vi "Measurement Logic.vi"() -> ()   [LabVIEW 2021, in "Line Transient Response with Pin Map.lvlib"]
uses:
  Line Transient Response with Pin Map.lvlib
  <vilib>/Plug-In SDKs/Measurements/Measure Call Context/Measure Call Context.lvclass
  Measurement Results.ctl
  Measurement Configuration.ctl
  <instrlib>/niScope/Controls/niScope vertical coupling.ctl
  subVIs/Reference values.ctl
  <vilib>/Plug-In SDKs/Clients/Session Management V1/Session Reservation/Session Reservation.lvclass
  common/builds/PMIC Common.lvlibp/Instrument Control/Scope/TClk/Instrument Info.ctl
  common/builds/PMIC Common.lvlibp/Instrument Control/Scope Parameters.ctl
  common/builds/PMIC Common.lvlibp/1abvi3w/instr.lib/niScope/Controls/niScope vertical coupling.ctl
  <instrlib>/niDCPower/nidcpower.llb/niDCPower Sense.ctl
  <instrlib>/niDCPower/nidcpower.llb/niDCPower Source Mode.ctl
  <instrlib>/niDCPower/nidcpower.llb/niDCPower Wait For Event - Event.ctl
  <instrlib>/niDCPower/nidcpower.llb/niDCPower Output Function.ctl
  <instrlib>/niDCPower/nidcpower.llb/niDCPower Aperture Time Units.ctl
  <vilib>/Plug-In SDKs/Measurements/Measure Call Context/Reserve Sessions - NPin.vi
  <vilib>/Plug-In SDKs/Sessions/niDCPower/Initialize Sessions - NSess.vi
  <vilib>/Plug-In SDKs/Sessions/niDCPower/Get Connections - 1Pin 1Conn.vi
  <instrlib>/niDCPower/nidcpower.llb/niDCPower Configure Digital Edge Measure Trigger With Channels.vi
  <instrlib>/niDCPower/nidcpower.llb/niDCPower Configure Digital Edge Source Trigger With Channels.vi
  <vilib>/Plug-In SDKs/Sessions/niScope/Initialize Sessions - NSess.vi
  <vilib>/Plug-In SDKs/Sessions/niScope/Get Connections - NPin MConn.vi
  <instrlib>/niScope/Configure/Trigger/niScope Configure Trigger Digital.vi
  <vilib>/Plug-In SDKs/Sessions/niDCPower/NI Session Management niDCPower.lvlib
  common/builds/PMIC Common.lvlibp
  <vilib>/Plug-In SDKs/Sessions/niScope/NI Session Management niScope.lvlib
panel:
  in  "measurement configuration":T1={"DUT setup time"=1.0, "Nominal output voltage"=3.3, "Source pin name"="", "Source current limit"=0.25, "Source maximum power"=300.0, "Source sample rate"=1800000.0, "Source voltage set point 1"=7.0, "Source voltage set point 2"=20.0, "Source voltatge pulse duration"=0.005, "Source voltage delay t1"=0.005, "Source voltage delay t2"=0.005, "Source voltage falling slew rate"=0.0055, "Source voltage rising slew rate"=24.0, "Source transient response"=1042, "Source voltage gain bandwidth"=2000.0, "Source voltage compensation frequency"=3530.0, "Source voltage pole-zero ratio"=2.0, "Load pin name"="", "Load voltage limit range"=4.0, "Load current level range"=4.0, "Load current level"=0.03, "Load transient response"=1042, "Load current gain bandwidth"=14000.0, "Load current compensation frequency"=180000.0, "Load current pole-zero ratio"=0.3, "Pin Names for Scope"=[], "vertical range"=[], "vertical offset"=[], "probe attenuation"=[], "vertical coupling"=[], "channel enabled"=[], "input impedance"=[], "max input frequency"=[], "min sample rate"=[], "reference position"=[], "min record length"=[], "enforce realtime"=[]} {"input impedance" items=["1 mega ohm"=0, "50 ohms"=2]; "vertical coupling" items=["AC", "DC", "Ground"]; "Source voltatge pulse duration" format="%#_6p"; "Source voltage rising slew rate" format="%#_6p"; "Load current pole-zero ratio" format="%#.2p"; "Load current compensation frequency" step=1000000.0 format="%#.2p"; "Load transient response" items=["Slow"=1041, "Normal"=1038, "Fast"=1039, "Custom"=1042]; "Source transient response" items=["Slow"=1041, "Normal"=1038, "Fast"=1039, "Custom"=1042]}
  out "measurement results":T3
  out "measure call context out":refnum<class "Measure Call Context.lvclass">
  in  "measure call context in":refnum<class "Measure Call Context.lvclass">
  out "error out":errorcluster
  in  "error in":errorcluster
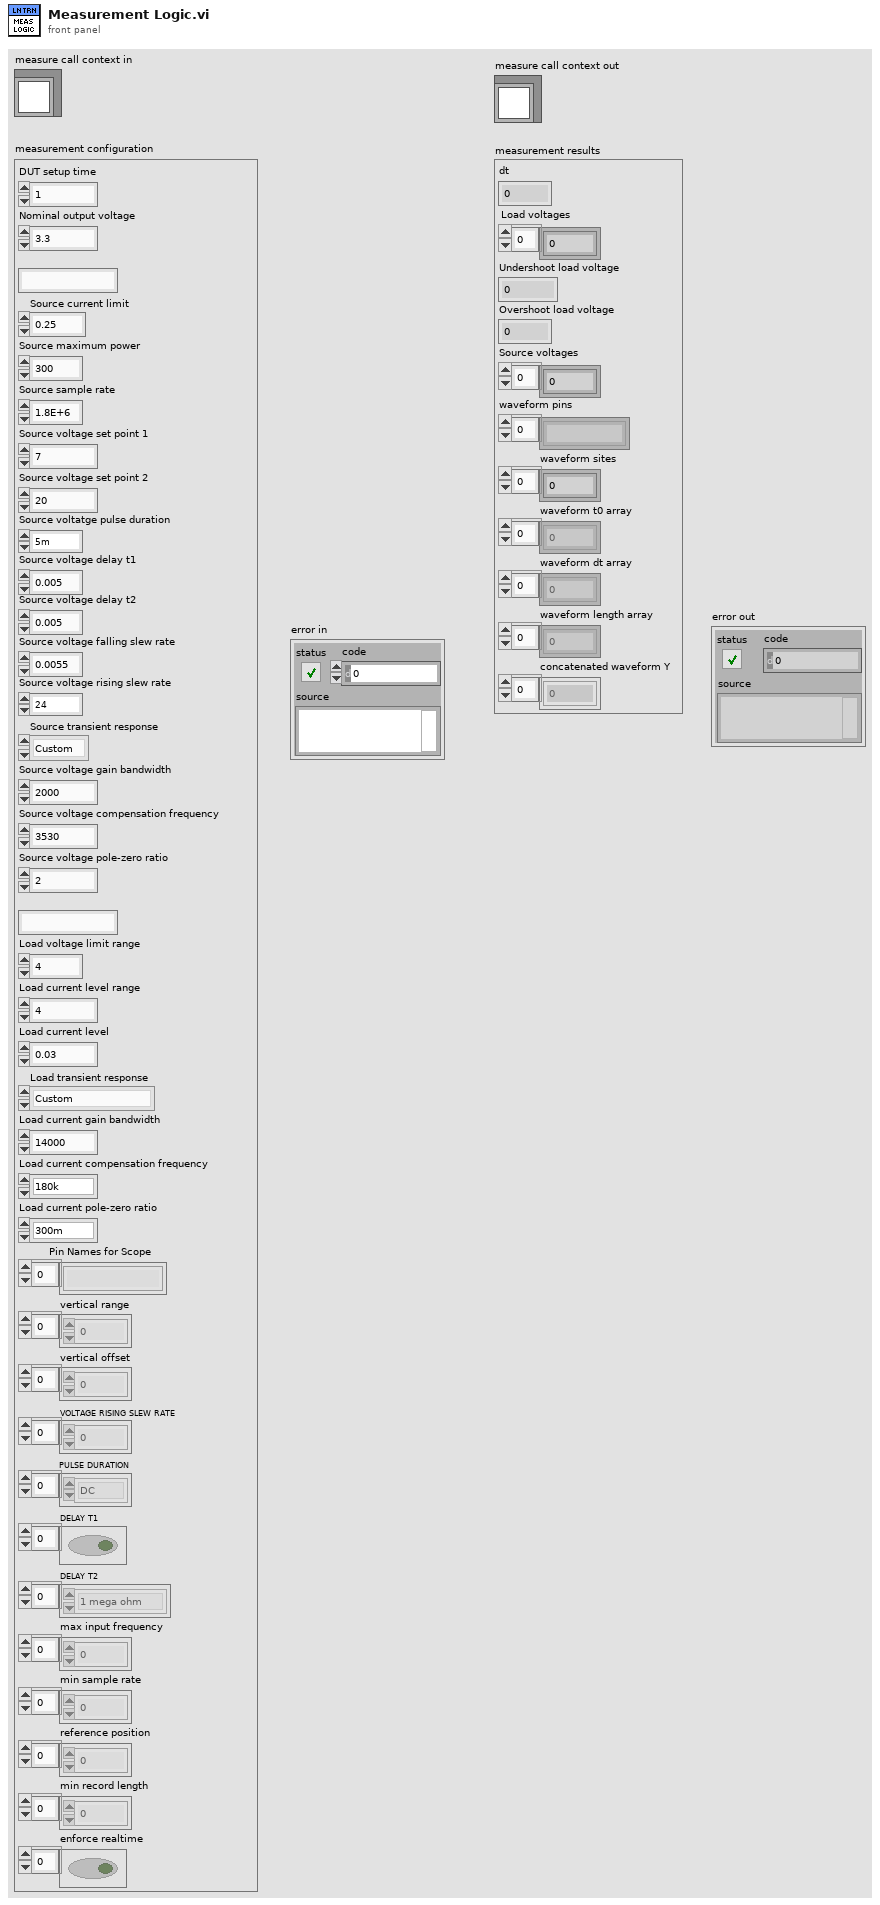
[diagram p1: front panel]
types:
  T1 = typedef "Line Transient Response with Pin Map.lvlib/Measurement Configuration.ctl" = cluster{"DUT setup time":dbl, "Nominal output voltage":dbl, "Source pin name":string, "Source current limit":dbl, "Source maximum power":dbl, "Source sample rate":dbl, "Source voltage set point 1":dbl, "Source voltage set point 2":dbl, "Source voltatge pulse duration":dbl, "Source voltage delay t1":dbl, "Source voltage delay t2":dbl, "Source voltage falling slew rate":dbl, "Source voltage rising slew rate":dbl, "Source transient response":i32, "Source voltage gain bandwidth":dbl, "Source voltage compensation frequency":dbl, "Source voltage pole-zero ratio":dbl, "Load pin name":string, "Load voltage limit range":dbl, "Load current level range":dbl, "Load current level":dbl, "Load transient response":i32, "Load current gain bandwidth":dbl, "Load current compensation frequency":dbl, "Load current pole-zero ratio":dbl, "Pin Names for Scope":string[], "vertical range":dbl[], "vertical offset":dbl[], "probe attenuation":dbl[], "vertical coupling":T2[], "channel enabled":bool[], "input impedance":u32[], "max input frequency":dbl[], "min sample rate":dbl[], "reference position":dbl[], "min record length":i32[], "enforce realtime":bool[]}
  T2 = typedef "niScope vertical coupling.ctl" = i32
  T3 = typedef "Line Transient Response with Pin Map.lvlib/Measurement Results.ctl" = cluster{"dt":dbl, "Load voltages":dbl[], "Undershoot load voltage":dbl, "Overshoot load voltage":dbl, "Source voltages":dbl[], "waveform pins":string[], "waveform sites":i32[], "waveform t0 array":dbl[], "waveform dt array":dbl[], "waveform length array":i32[], "concatenated waveform Y":dbl[]}
  T4 = typedef "Line Transient Response with Pin Map.lvlib/Reference values.ctl" = cluster{"dcpower session reservation":refnum<class "Session Reservation.lvclass">, "Source out":refnum<k15>, "Source channel name":string, "Load out":refnum<k15>, "Load channel name":string, "Scope out":refnum<k15>, "Scope channel name":string, "Source sequence name":string, "Source terminal name":string, "Start source terminal name":string, "Measure load terminal name":string, "Scope ref trigger source":string, "Measure record length smu":i32, "Aperture time":dbl, "Measure record length scope":i32, "scope session reservation":refnum<class "Session Reservation.lvclass">, "Scope handles":refnum<k15>[][], "connection map":map{string, T5[]}, "instrument info map array":map{string, cluster{"channel":string, "siteNumber":i32, "pin":string, "Scope Parameters":T6}[]}[], "Enable TClk":bool, "Number of records":i32, "measurement results":T3}
  T5 = typedef "PMIC Common.lvlibp/Instrument Info.ctl" = cluster{"instrument":string, "channel":string, "siteNumber":i32}
  T6 = typedef "PMIC Common.lvlibp/Scope Parameters.ctl" = cluster{"vertical range":dbl, "vertical offset":dbl, "probe attenuation":dbl, "vertical coupling":T7, "channel enabled":bool, "input impedance":u32, "maximum input frequency":dbl, "min sample rate":dbl, "reference position":dbl, "min record length":i32, "number of records":i32, "enforce realtime":bool}
  T7 = typedef "PMIC Common.lvlibp/niScope vertical coupling.ctl" = i32
  T8 = typedef "niDCPower Wait For Event - Event.ctl" = i32
  T9 = typedef "niDCPower Source Mode.ctl" = i32
  T10 = typedef "niDCPower Sense.ctl" = i32
  T11 = typedef "NI Session Management niDCPower.lvlib/Connection with Session.ctl" = cluster{"connection":T12, "session":refnum<k15>}
  T12 = typedef "NI Session Management V1 Client.lvlib/Session Reservation.lvclass/Connection.ctl" = cluster{"pin or relay name":string, "site":i32, "instrument type id":string, "channel":string}
  T13 = typedef "niDCPower Aperture Time Units.ctl" = i32
  T14 = typedef "niDCPower Output Function.ctl" = i32
  T15 = cluster{"Numeric":dbl, "Numeric":dbl, "Numeric":dbl, "vertical coupling":T2, "Boolean":bool, "input impedance":u32, "Numeric":dbl, "Numeric":dbl, "Numeric":dbl, "Numeric":i32, "Number of records":i32, "Boolean":bool}[]
  T16 = typedef "NI Session Management niScope.lvlib/Connection with Session.ctl" = cluster{"connection":T12, "session":refnum<k15>}
  T17 = typedef "NI Measurement Plug-In SDK.lvlib/Pin Map Context.ctl" = cluster{"pin map id":string, "sites":i32[]}
  T18 = map{string, cluster{"channel":string, "siteNumber":i32, "pin":string, "Scope Parameters":T6}[]}[]
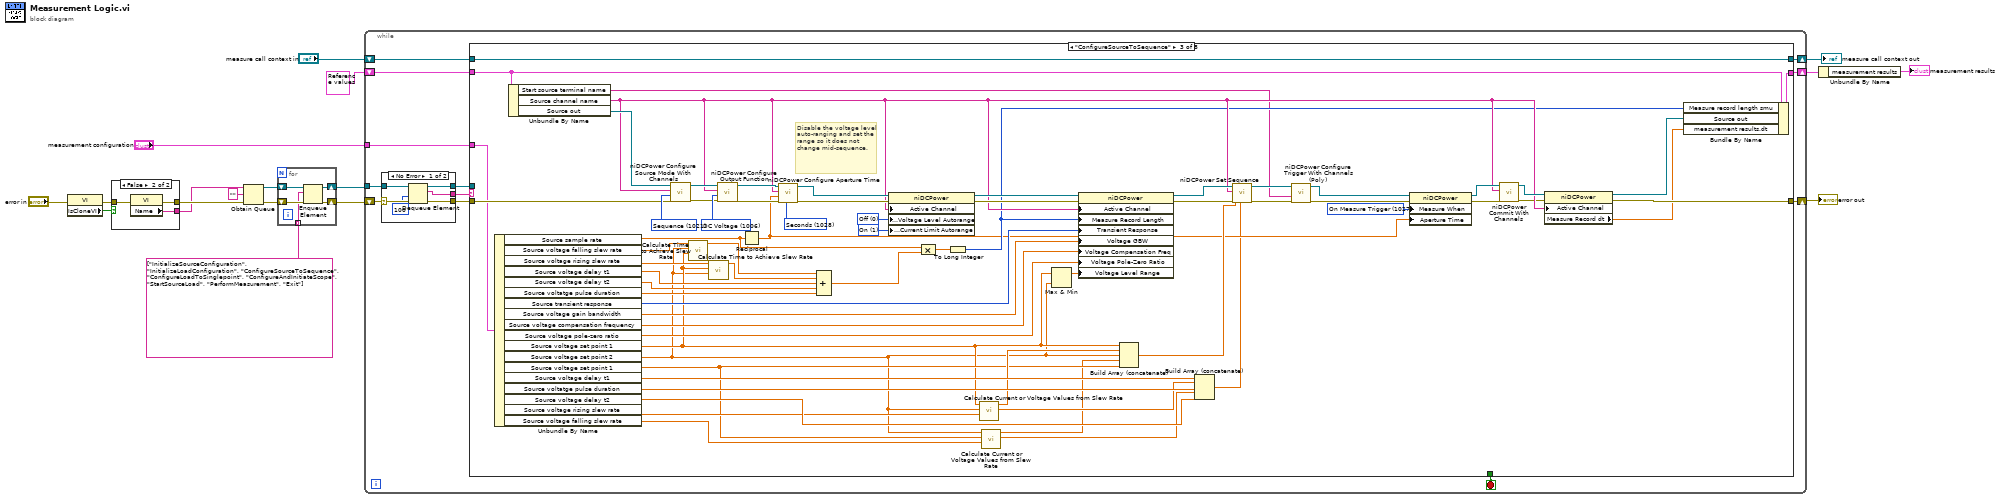
[diagram p0: block diagram]
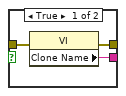
[diagram p2: hidden frame]
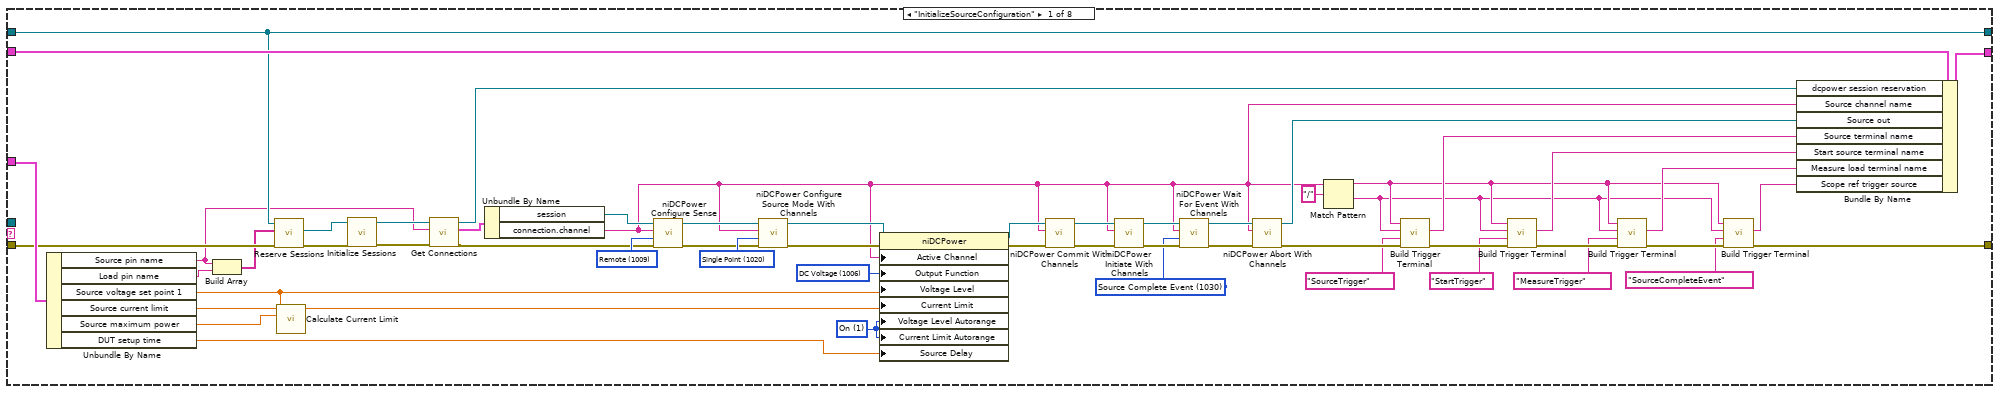
[diagram p3: hidden frame]
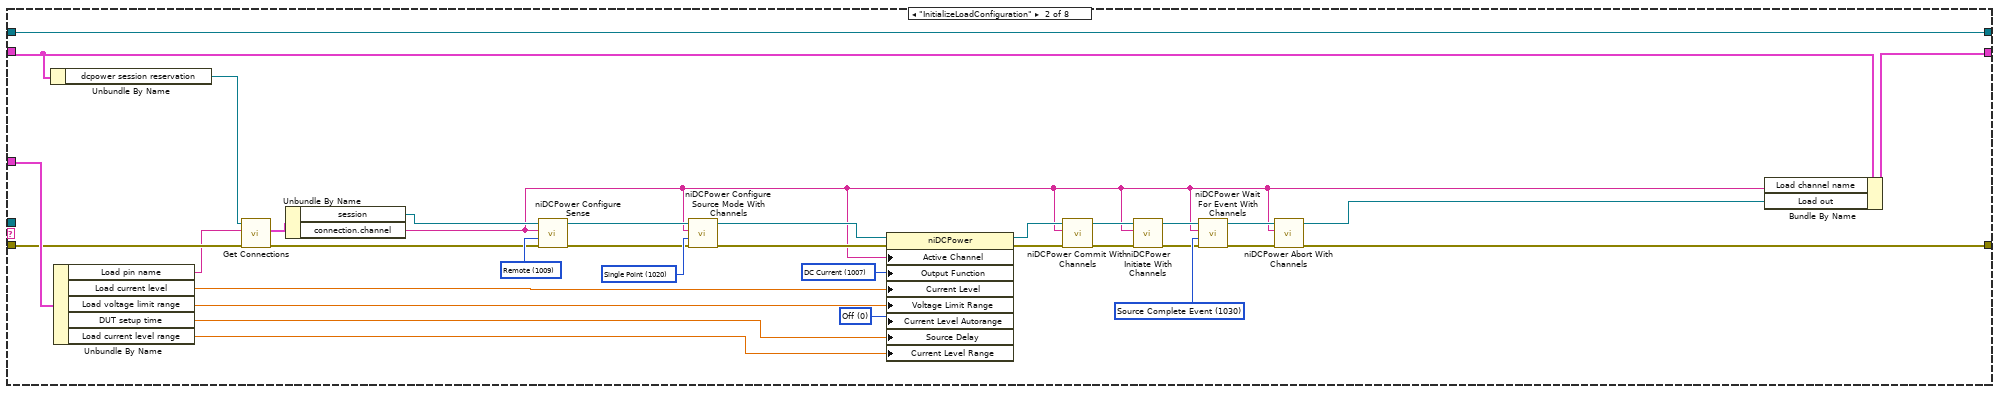
[diagram p4: hidden frame]
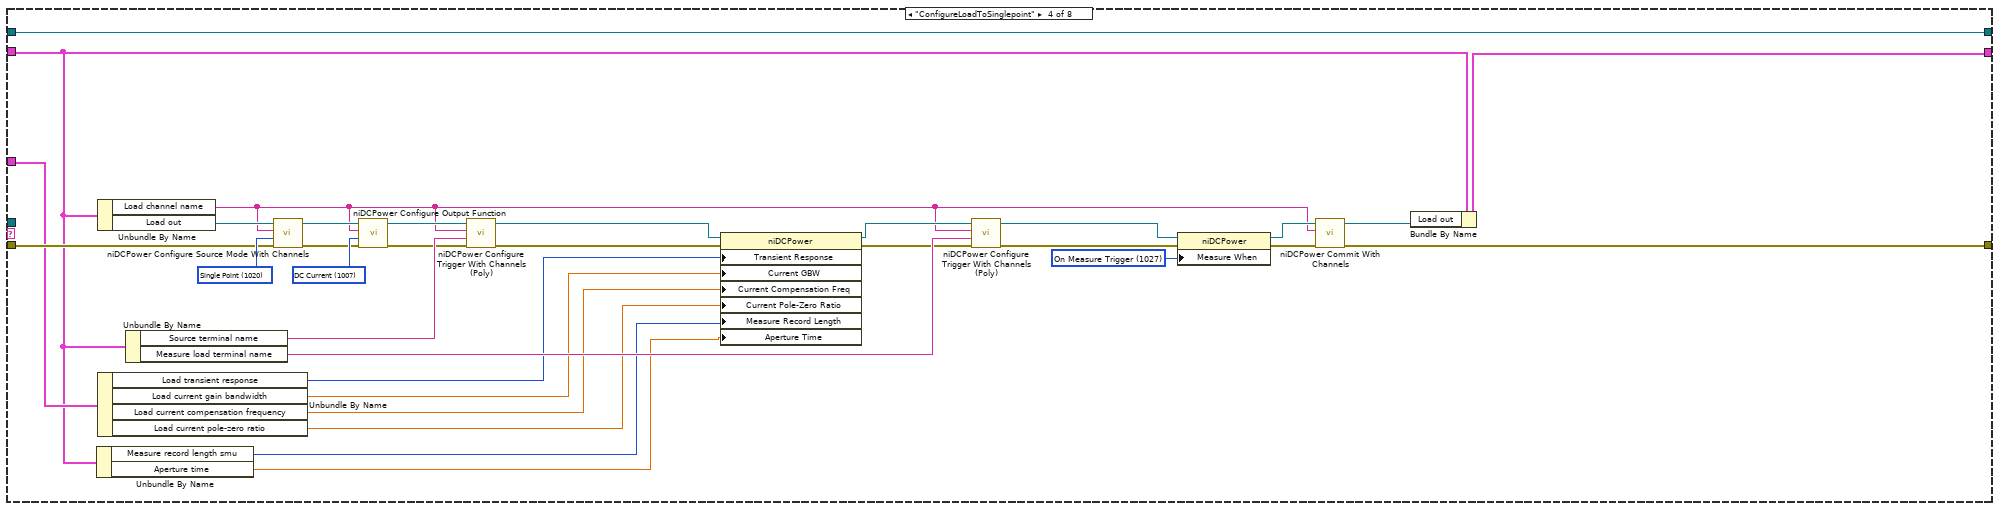
[diagram p5: hidden frame]
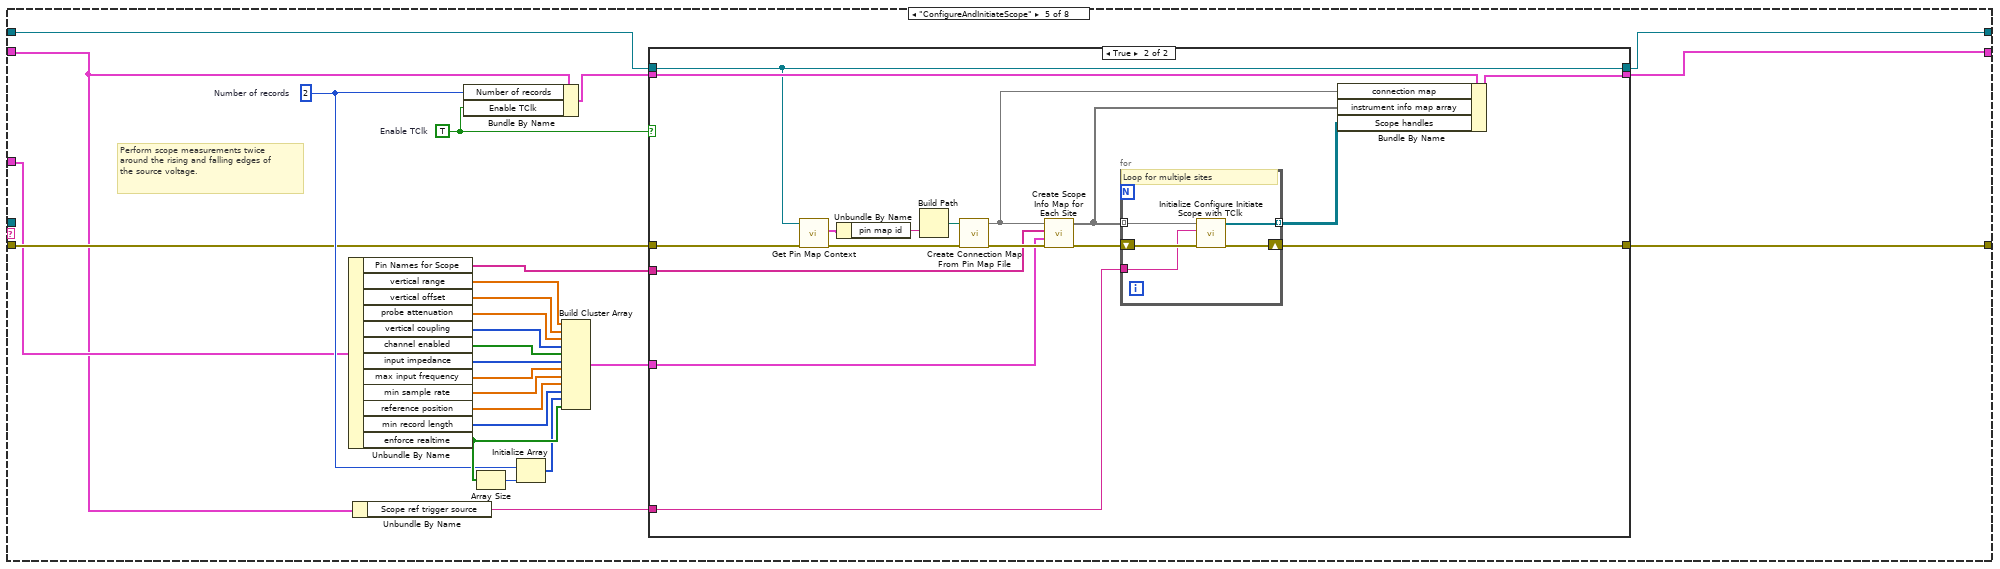
[diagram p6: hidden frame]
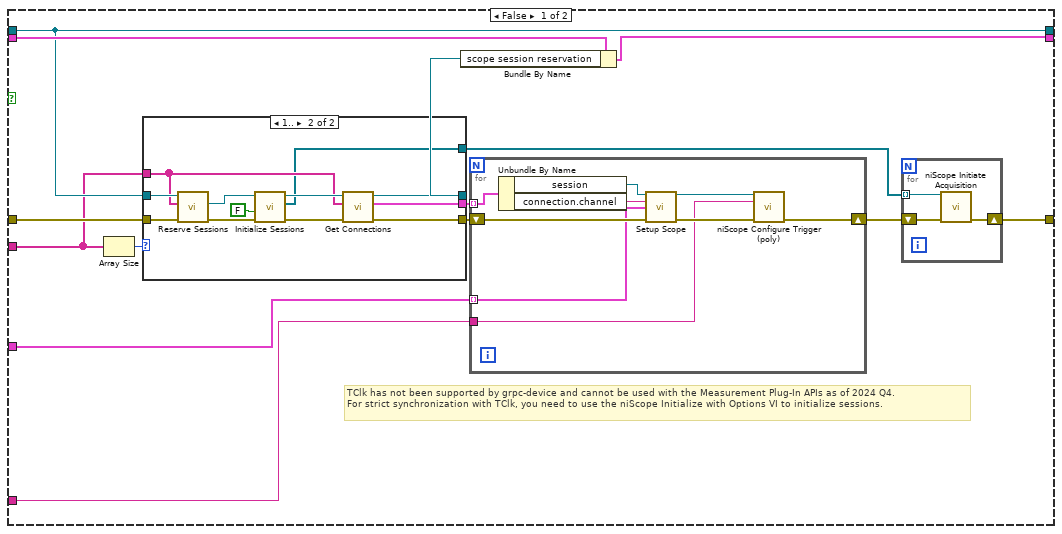
[diagram p7: hidden frame]
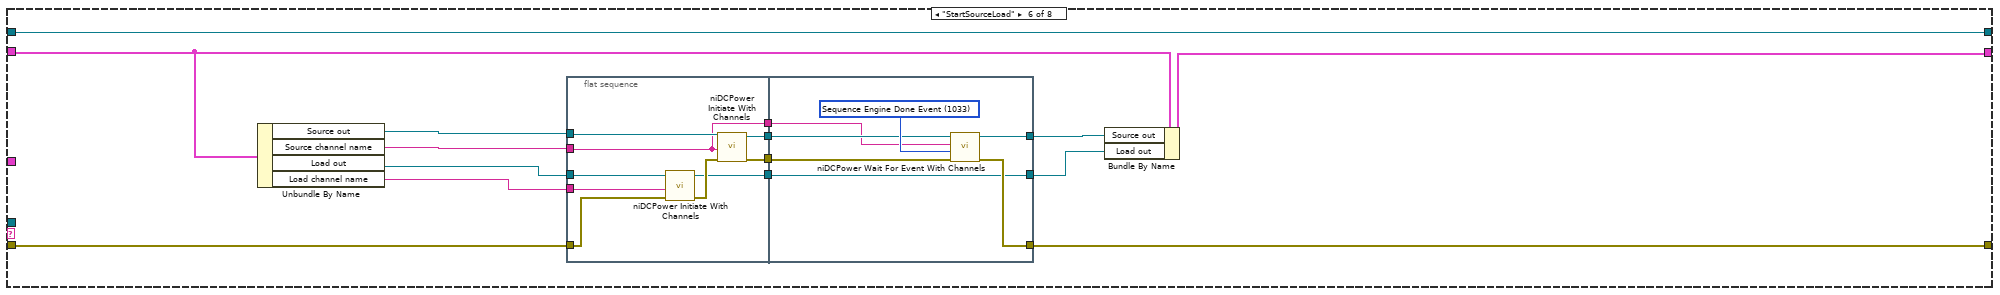
[diagram p9: hidden frame]
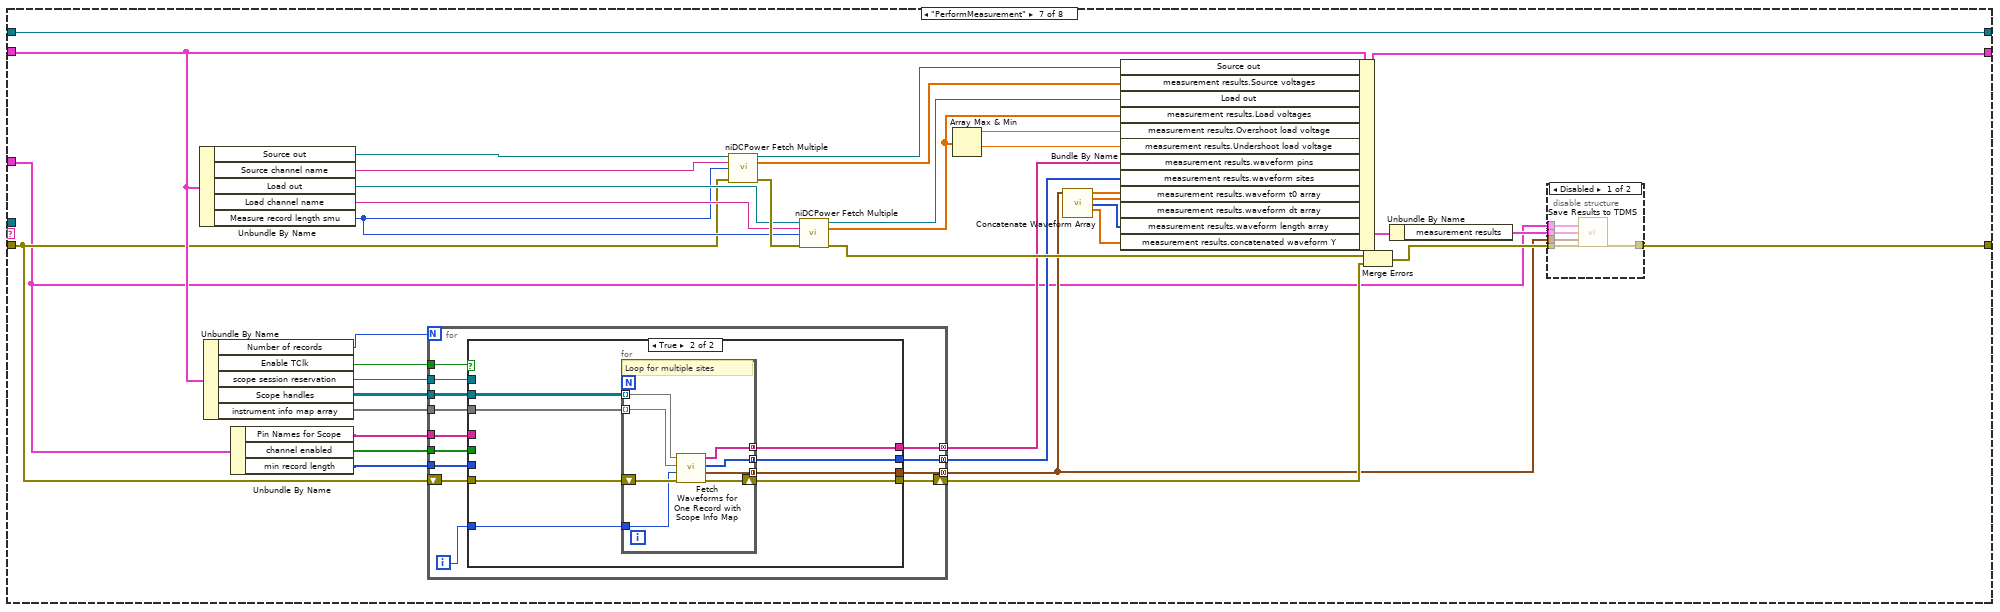
[diagram p10: hidden frame]
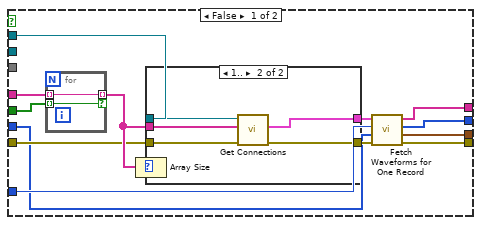
[diagram p12: hidden frame]
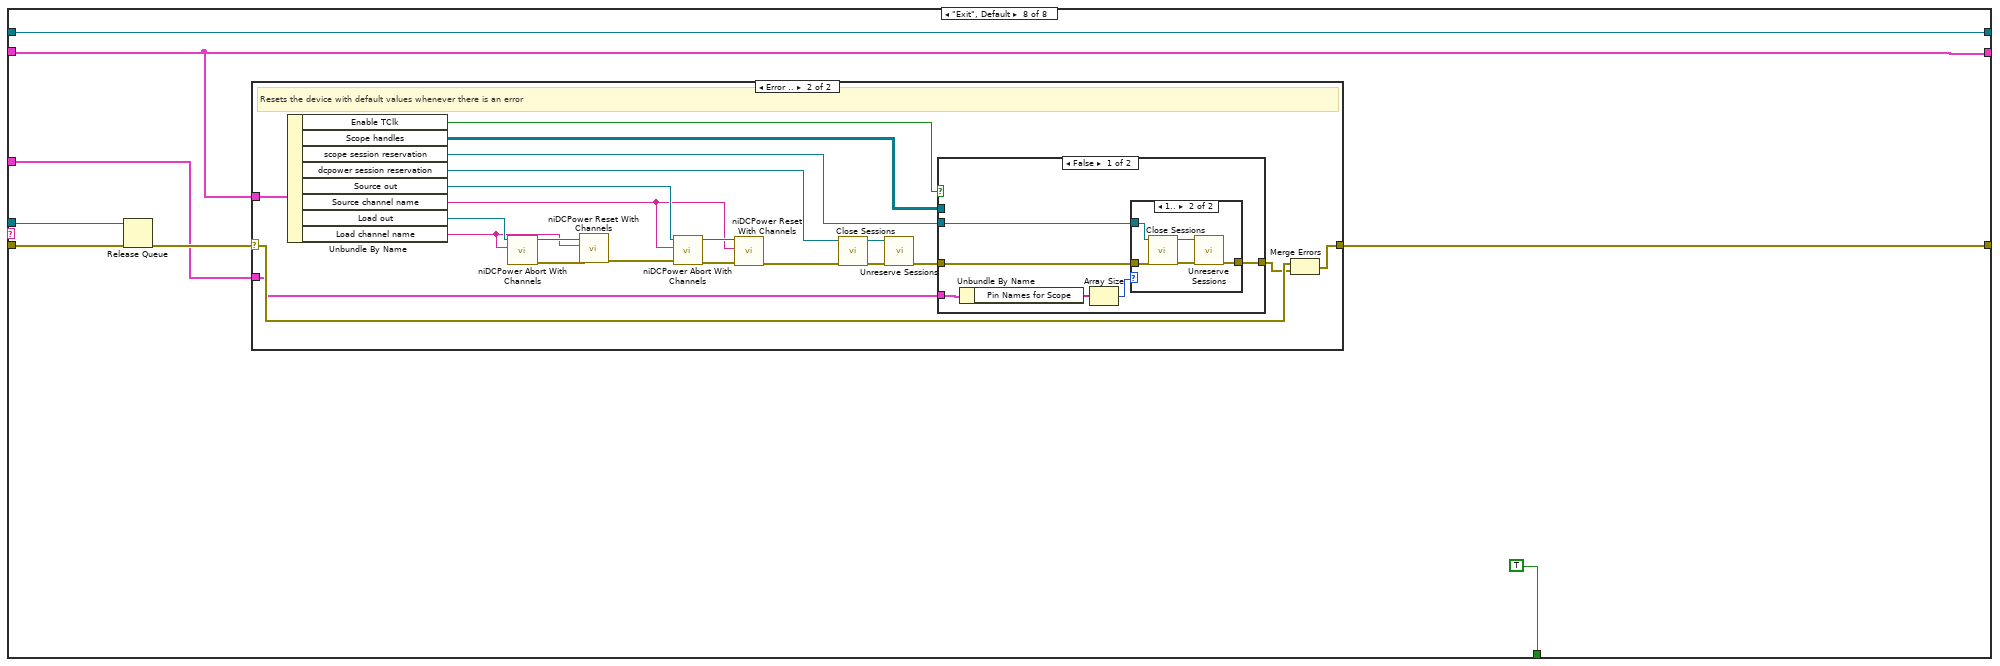
[diagram p14: hidden frame]
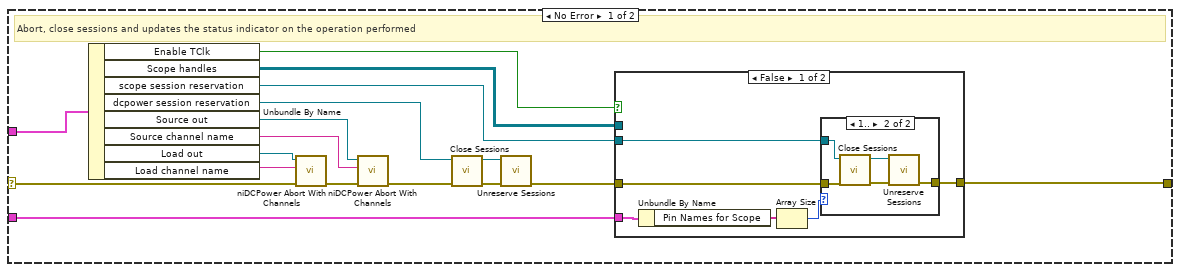
[diagram p15: hidden frame]
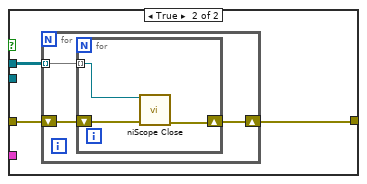
[diagram p17: hidden frame]
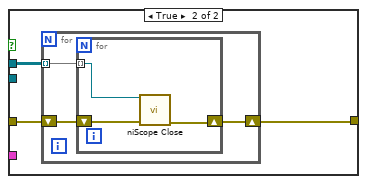
[diagram p19: hidden frame]
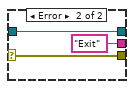
[diagram p20: hidden frame]
diagram:
  n1 = property class="VI"(error in="error in") -> (error out=w17:errorcluster, "IsCloneVI"=w18:bool)  [unwired: 1 in, 1 out]
  n2 = case shown="False" w18 {
    tunnel: [w21 w24] -> w16
    tunnel: [w20 w23] -> w15
    tunnel: w17 -> [w19 w22]
    frame True {
      n3 = property class="VI"(error in=w19) -> (error out=w21:errorcluster, "Clone Name"=w20:string)  [unwired: 1 in, 1 out]
    }
    frame False {
      n4 = property class="VI"(error in=w22) -> (error out=w24:errorcluster, "Name"=w23:string)  [unwired: 1 in, 1 out]
    }
  }
  n5 = Obtain Queue(name (unnamed)=w15, element data type="", error in (no error)=w16) -> (queue out=w13:refnum<queue>, error out=w14:errorcluster)  [unwired: 2 in, 1 out]
  n6 = for {
    shift-right: [w27] -> w10
    shift-left: w13 -> [w29]
    shift-right: [w26] -> w9
    shift-left: w14 -> [w28]
    tunnel: string[] ["InitializeSourceConfiguration", "InitializeLoadConfiguration", "ConfigureSourceToSequence", "ConfigureLoadToSinglepoint", "ConfigureAndInitiateScope", "StartSourceLoad", "PerformMeasurement", "Exit"] ("Step sequence") -> [w25] mode=indexing
    n7 = Enqueue Element(queue=w29, element=w25, error in (no error)=w28) -> (queue out=w27:refnum<queue>, error out=w26:errorcluster)  [unwired: 1 in, 1 out]
  }
  n8 = while {
    tunnel: w10 -> [w41]
    shift-right: [w34] -> w7
    shift-left: w9 -> [w40]
    tunnel: "measurement configuration" -> [w38]
    shift-right: [w36] -> w6
    shift-left: T4 {"dcpower session reservation"=refnum, "Source out"="", "Source channel name"="", "Load out"="", "Load channel name"="", "Scope out"="", "Scope channel name"="", "Source sequence name"="", "Source terminal name"="", "Start source terminal name"="", "Measure load terminal name"="", "Scope ref trigger source"="", "Measure record length smu"=0, "Aperture time"=0.0, "Measure record length scope"=0, "scope session reservation"=refnum, "Scope handles"=[], "connection map"={}, "instrument info map array"=[], "Enable TClk"=FALSE, "Number of records"=2, "measurement results"={"dt"=0.0, "Load voltages"=[0.0], "Undershoot load voltage"=0.0, "Overshoot load voltage"=0.0, "Source voltages"=[0.0], "waveform pins"=[], "waveform sites"=[0], "waveform t0 array"=[], "waveform dt array"=[], "waveform length array"=[], "concatenated waveform Y"=[]}} -> [w37]
    shift-right: [w32] -> w4
    shift-left: "measure call context in" -> [w31]
    stop <- w33 stop-if-true
    n9 = case shown="No Error" w40 {
      selector: w40 -> [w534 w538]
      tunnel: w41 -> [w536 w537]
      tunnel: [w535 "Exit" ("t")] -> w39
      tunnel: [w533 w538] -> w35
      tunnel: [w531 w537] -> w30
      frame No Error {
        n10 = Dequeue Element(queue=w536, timeout in ms (-1)=100, error in (no error)=w534) -> (queue out=w531:refnum<queue>, element=w535:string, error out=w533:errorcluster)  [unwired: 1 out]
      }
      frame Error {
      }
    }
    n11 = case shown="\"ConfigureSourceToSequence\"" w39 {
      tunnel: w38 -> [w79 w109 w169 w211 w234 _ w348 w445]
      tunnel: w37 -> [w54 w100 w167 w207 w231 w320 w362 w444]
      tunnel: [w78 w108 w166 w205 w230 w319 w350 w444] -> w36
      tunnel: w35 -> [w57 w104 w170 w213 w236 w321 w361 w446]
      tunnel: [w46 w106 w165 w208 w235 w318 w352 w443] -> w34
      tunnel: [_ _ _ _ _ _ _ TRUE] -> w33
      tunnel: [w53 w107 w164 w204 w232 w317 w384 w448] -> w32
      tunnel: w31 -> [w53 w107 w164 w204 w233 w317 w384 w448]
      tunnel: w30 -> [_ _ _ _ _ _ _ w442]
      frame "InitializeSourceConfiguration" {
        w81 = 1 items=["Off", "On"] ("Source:DC Voltage:Voltage Level Autorange")
        w82 = T8 1030 items=["Source Complete Event"=1030, "Measure Complete Event"=1031, "Sequence Iteration Complete Event"=1032, "Sequence Engine Done Event"=1033, "Pulse Complete Event"=1051, "Ready For Pulse Trigger Event"=1052] ("event")
        w93 = T9 1020 items=["Single Point"=1020, "Sequence"=1021] ("source mode")
        w88 = 1006 items=["DC Voltage"=1006, "DC Current"=1007, "Pulse Voltage"=1049, "Pulse Current"=1050] ("Source:Output Function")
        w83 = T10 1009 items=["Local"=1008, "Remote"=1009] ("sense")
        n12 = Unbundle By Name(w79) -> ("Source pin name"=w52:string, "Load pin name"=w58:string, "Source voltage set point 1"=w73:dbl, "Source current limit"=w70:dbl, "Source maximum power"=w71:dbl, "DUT setup time"=w74:dbl)
        n13 = Build Array(w52, w58) -> (w55:string[])
        n14 = call-poly <vilib>:"Reserve Sessions.vi"("error in"=w57, "pin or relay names"=w55, "measurement context in"=w53) -> ("error out"=w63:errorcluster, "session reservation out"=w62:refnum<class "Session Reservation.lvclass">)  [unwired: 6 in, 1 out]
        n15 = call "Calculate Current Limit.vi"("Voltage value"=w73, "Maximum power"=w71, "Current limit in"=w70) -> ("Current limit out"=w72:dbl)  [unwired: 8 in]
        n16 = call-poly <vilib>:"Initialize Sessions.vi"("error in"=w63, "session reservation in"=w62) -> ("error out"=w61:errorcluster, "session reservation out"=w60:refnum<class "Session Reservation.lvclass">)  [unwired: 6 in, 2 out]
        n17 = call-poly <vilib>:"Get Connections.vi"("error in"=w61, "pin or relay name"=w52, "session reservation in"=w60) -> ("error out"=w56:errorcluster, "connection"=w59:T11, "session reservation out"=w48:refnum<class "Session Reservation.lvclass">)  [unwired: 6 in]
        n18 = Unbundle By Name(w59) -> ("session"=w51:refnum<k15>, "connection.channel"=w49:string)
        n19 = call <instrlib>:"niDCPower Configure Sense.vi"("error in (no error)"=w56, "sense"=w83, "channel name"=w49, "instrument handle"=w51) -> ("error out"=w91:errorcluster, "instrument handle out"=w89:refnum<k15>)  [unwired: 6 in]
        n20 = call <instrlib>:"niDCPower Configure Source Mode With Channels.vi"("error in (no error)"=w91, "source mode"=w93, "channel name"=w49, "instrument handle"=w89) -> ("error out"=w92:errorcluster, "instrument handle out"=w90:refnum<k15>)  [unwired: 6 in]
        n21 = property class="niDCPower"(reference=w90, error in=w92, "Active Channel"=w49, "Output Function"=w88, "Voltage Level"=w73, "Current Limit"=w72, "Voltage Level Autorange"=w81, "Current Limit Autorange"=w81, "Source Delay"=w74) -> (reference out=w94:refnum<k15>, error out=w95:errorcluster)
        n22 = call <instrlib>:"niDCPower Commit With Channels.vi"("error in (no error)"=w95, "channel name"=w49, "instrument handle"=w94) -> ("error out"=w97:errorcluster, "instrument handle out"=w96:refnum<k15>)  [unwired: 7 in]
        n23 = call <instrlib>:"niDCPower Initiate With Channels.vi"("error in (no error)"=w97, "channel name"=w49, "instrument handle"=w96) -> ("error out"=w84:errorcluster, "instrument handle out"=w85:refnum<k15>)  [unwired: 7 in]
        n24 = call <instrlib>:"niDCPower Wait For Event With Channels.vi"("error in (no error)"=w84, "event"=w82, "channel name"=w49, "instrument handle"=w85) -> ("error out"=w87:errorcluster, "instrument handle out"=w86:refnum<k15>)  [unwired: 6 in]
        n25 = call <instrlib>:"niDCPower Abort With Channels.vi"("error in (no error)"=w87, "channel name"=w49, "instrument handle"=w86) -> ("error out"=w77:errorcluster, "instrument handle out"=w80:refnum<k15>)  [unwired: 7 in]
        n26 = Match Pattern(string=w49, regular expression="/") -> (before substring=w44:string, after substring=w43:string)  [unwired: 1 in, 2 out]
        n27 = call "Build Trigger Terminal.vi"("error in (no error)"=w77, "Trigger/Event Name"="SourceTrigger", "Channel Name"=w43, "Resource Name"=w44) -> ("error out"=w75:errorcluster, "Terminal Name"=w64:string)  [unwired: 6 in]
        n28 = call "Build Trigger Terminal.vi"("error in (no error)"=w75, "Trigger/Event Name"="StartTrigger", "Channel Name"=w43, "Resource Name"=w44) -> ("error out"=w67:errorcluster, "Terminal Name"=w68:string)  [unwired: 6 in]
        n29 = call "Build Trigger Terminal.vi"("error in (no error)"=w67, "Trigger/Event Name"="MeasureTrigger", "Channel Name"=w43, "Resource Name"=w44) -> ("error out"=w47:errorcluster, "Terminal Name"=w65:string)  [unwired: 6 in]
        n30 = call "Build Trigger Terminal.vi"("error in (no error)"=w47, "Trigger/Event Name"="SourceCompleteEvent", "Channel Name"=w43, "Resource Name"=w44) -> ("error out"=w46:errorcluster, "Terminal Name"=w42:string)  [unwired: 6 in]
        n31 = Bundle By Name(cluster=w54, "dcpower session reservation"=w48, "Source channel name"=w49, "Source out"=w80, "Source terminal name"=w64, "Start source terminal name"=w68, "Measure load terminal name"=w65, "Scope ref trigger source"=w42) -> (w78:T4)
      }
      frame "InitializeLoadConfiguration" {
        w127 = T9 1020 items=["Single Point"=1020, "Sequence"=1021] ("source mode")
        w120 = T8 1030 items=["Source Complete Event"=1030, "Measure Complete Event"=1031, "Sequence Iteration Complete Event"=1032, "Sequence Engine Done Event"=1033, "Pulse Complete Event"=1051, "Ready For Pulse Trigger Event"=1052] ("event")
        w115 = 0 items=["Off", "On"] ("Source:DC Current:Current Level Autorange")
        w117 = 1007 items=["DC Voltage"=1006, "DC Current"=1007, "Pulse Voltage"=1049, "Pulse Current"=1050] ("Source:Output Function")
        w116 = T10 1009 items=["Local"=1008, "Remote"=1009] ("sense")
        n32 = Unbundle By Name(w100) -> ("dcpower session reservation"=w99:refnum<class "Session Reservation.lvclass">)
        n33 = Unbundle By Name(w109) -> ("Load pin name"=w101:string, "Load current level"=w112:dbl, "Load voltage limit range"=w111:dbl, "DUT setup time"=w114:dbl, "Load current level range"=w110:dbl)
        n34 = call-poly <vilib>:"Get Connections.vi"("error in"=w104, "pin or relay name"=w101, "session reservation in"=w99) -> ("error out"=w103:errorcluster, "connection"=w105:T11)  [unwired: 6 in, 1 out]
        n35 = Unbundle By Name(w105) -> ("session"=w102:refnum<k15>, "connection.channel"=w98:string)
        n36 = call <instrlib>:"niDCPower Configure Sense.vi"("error in (no error)"=w103, "sense"=w116, "channel name"=w98, "instrument handle"=w102) -> ("error out"=w124:errorcluster, "instrument handle out"=w123:refnum<k15>)  [unwired: 6 in]
        n37 = call <instrlib>:"niDCPower Configure Source Mode With Channels.vi"("error in (no error)"=w124, "source mode"=w127, "channel name"=w98, "instrument handle"=w123) -> ("error out"=w126:errorcluster, "instrument handle out"=w125:refnum<k15>)  [unwired: 6 in]
        n38 = property class="niDCPower"(reference=w125, error in=w126, "Active Channel"=w98, "Output Function"=w117, "Current Level"=w112, "Voltage Limit Range"=w111, "Current Level Autorange"=w115, "Source Delay"=w114, "Current Level Range"=w110) -> (reference out=w128:refnum<k15>, error out=w129:errorcluster)
        n39 = call <instrlib>:"niDCPower Commit With Channels.vi"("error in (no error)"=w129, "channel name"=w98, "instrument handle"=w128) -> ("error out"=w130:errorcluster, "instrument handle out"=w131:refnum<k15>)  [unwired: 7 in]
        n40 = call <instrlib>:"niDCPower Initiate With Channels.vi"("error in (no error)"=w130, "channel name"=w98, "instrument handle"=w131) -> ("error out"=w118:errorcluster, "instrument handle out"=w119:refnum<k15>)  [unwired: 7 in]
        n41 = call <instrlib>:"niDCPower Wait For Event With Channels.vi"("error in (no error)"=w118, "event"=w120, "channel name"=w98, "instrument handle"=w119) -> ("error out"=w122:errorcluster, "instrument handle out"=w121:refnum<k15>)  [unwired: 6 in]
        n42 = call <instrlib>:"niDCPower Abort With Channels.vi"("error in (no error)"=w122, "channel name"=w98, "instrument handle"=w121) -> ("error out"=w106:errorcluster, "instrument handle out"=w113:refnum<k15>)  [unwired: 7 in]
        n43 = Bundle By Name(cluster=w100, "Load channel name"=w98, "Load out"=w113) -> (w108:T4)
      }
      frame "ConfigureSourceToSequence" {
        w135 = 0 items=["Off", "On"] ("Source:DC Voltage:Voltage Level Autorange")
        w182 = T13 1028 items=["Seconds"=1028, "Powerline Cycles"=1029] ("aperture time units")
        w189 = 1027 items=["Automatically after Source Complete"=1025, "On Demand"=1026, "On Measure Trigger"=1027] ("Measurement:Advanced:Measure When")
        w194 = 1 items=["Off", "On"] ("DC Voltage:Voltage Level Autorange")
        w193 = T14 1006 items=["DC Voltage"=1006, "DC Current"=1007, "Pulse Voltage"=1049, "Pulse Current"=1050] ("output function")
        w192 = T9 1021 items=["Single Point"=1020, "Sequence"=1021] ("source mode")
        # "Disable the voltage level auto-ranging and set the range so it does not change mid-sequence."
        n44 = Unbundle By Name(w169) -> ("Source sample rate"=w149:dbl, "Source voltage falling slew rate"=w147:dbl, "Source voltage rising slew rate"=w145:dbl, "Source voltage delay t1"=w162:dbl, "Source voltage delay t2"=w148:dbl, "Source voltatge pulse duration"=w160:dbl, "Source transient response"=w168:i32, "Source voltage gain bandwidth"=w181:dbl, "Source voltage compensation frequency"=w180:dbl, "Source voltage pole-zero ratio"=w179:dbl, "Source voltage set point 1"=w133:dbl, "Source voltage set point 2"=w132:dbl, "Source voltage set point 1"=w140:dbl, "Source voltage delay t1"=w153:dbl, "Source voltatge pulse duration"=w151:dbl, "Source voltage delay t2"=w150:dbl, "Source voltage rising slew rate"=w143:dbl, "Source voltage falling slew rate"=w139:dbl)
        n45 = Unbundle By Name(w167) -> ("Start source terminal name"=w154:string, "Source channel name"=w172:string, "Source out"=w197:refnum<k15>)
        n46 = call <instrlib>:"niDCPower Configure Source Mode With Channels.vi"("error in (no error)"=w170, "source mode"=w192, "channel name"=w172, "instrument handle"=w197) -> ("error out"=w190:errorcluster, "instrument handle out"=w191:refnum<k15>)  [unwired: 6 in]
        n47 = call "Calculate Time to Achieve Slew Rate.vi"("Current/voltage set point 2"=w133, "Current/voltage set point 1"=w132, "Current/voltage slew rate"=w147) -> ("Calculated time"=w146:dbl)  [unwired: 8 in]
        n48 = call "Calculate Time to Achieve Slew Rate.vi"("Current/voltage set point 2"=w132, "Current/voltage set point 1"=w133, "Current/voltage slew rate"=w145) -> ("Calculated time"=w144:dbl)  [unwired: 8 in]
        n49 = call <instrlib>:"niDCPower Configure Output Function.vi"("error in (no error)"=w190, "output function"=w193, "channel name"=w172, "instrument handle"=w191) -> ("error out"=w186:errorcluster, "instrument handle out"=w184:refnum<k15>)  [unwired: 6 out]
        n50 = Reciprocal(x=w149) -> (1/x=w159:dbl)
        n51 = call <instrlib>:"niDCPower Configure Aperture Time.vi"("aperture time units"=w182, "error in (no error)"=w186, "aperture time"=w159, "channel name"=w172, "instrument handle"=w184) -> ("error out"=w185:errorcluster, "instrument handle out"=w183:refnum<k15>)  [unwired: 5 in]
        n52 = Compound Arithmetic op=ADD(w146, w144, w162, w148, w160) -> (w161:dbl)
        n53 = property class="niDCPower"(reference=w183, error in=w185, "Active Channel"=w172, "Source:DC Voltage:Voltage Level Autorange"=w135, "Source:DC Voltage:Current Limit Autorange"=w194) -> (reference out=w195:refnum<k15>, error out=w196:errorcluster)
        n54 = Compound Arithmetic op=MULTIPLY(w149, w161) -> (w178:dbl)
        n55 = To Long Integer(number=w178) -> (32bit integer=w163:i32)
        n56 = call "Calculate Current or Voltage Values from Slew Rate.vi"("Current/voltage slew rate"=w143, "Current/voltage end point"=w132, "Current/voltage start point"=w133) -> ("Source delays"=w141:dbl[], "Current/voltage values"=w142:dbl[])  [unwired: 7 in]
        n57 = call "Calculate Current or Voltage Values from Slew Rate.vi"("Current/voltage slew rate"=w139, "Current/voltage end point"=w140, "Current/voltage start point"=w132) -> ("Source delays"=w137:dbl[], "Current/voltage values"=w138:dbl[])  [unwired: 7 in]
        n58 = Max & Min(x=w133, y=w132) -> (max(x,y)=w134:dbl)  [unwired: 1 out]
        n59 = property class="niDCPower"(reference=w195, error in=w196, "Active Channel"=w172, "Measure Record Length"=w163, "Transient Response"=w168, "Voltage GBW"=w181, "Voltage Compensation Freq"=w180, "Voltage Pole-Zero Ratio"=w179, "Voltage Level Range"=w134) -> (reference out=w176:refnum<k15>, error out=w177:errorcluster)
        n60 = Build Array (concatenate)(w133, w142, w132, w138, w140) -> (w175:dbl[])
        n61 = Build Array (concatenate)(w153, w141, w151, w137, w150) -> (w152:dbl[])
        n62 = call <instrlib>:"niDCPower Set Sequence.vi"("source delays"=w152, "error in (no error)"=w177, "values"=w175, "channel name"=w172, "instrument handle"=w176) -> ("error out"=w157:errorcluster, "instrument handle out"=w158:refnum<k15>)  [unwired: 5 in]
        n63 = call-poly <instrlib>:"niDCPower Configure Trigger With Channels (Poly).vi"("error in (no error)"=w157, "input terminal"=w154, "instrument handle"=w158) -> ("error out"=w155:errorcluster, "instrument handle out"=w156:refnum<k15>)  [unwired: 7 in]
        n64 = property class="niDCPower"(reference=w156, error in=w155, "Measure When"=w189, "Aperture Time"=w159) -> (reference out=w187:refnum<k15>, error out=w188:errorcluster)
        n65 = call <instrlib>:"niDCPower Commit With Channels.vi"("error in (no error)"=w188, "channel name"=w172, "instrument handle"=w187) -> ("error out"=w171:errorcluster, "instrument handle out"=w174:refnum<k15>)  [unwired: 7 in]
        n66 = property class="niDCPower"(reference=w174, error in=w171, "Active Channel"=w172) -> (reference out=w173:refnum<k15>, error out=w165:errorcluster, "Measure Record dt"=w136:dbl)
        n67 = Bundle By Name(cluster=w167, "Measure record length smu"=w163, "Source out"=w173, "measurement results.dt"=w136) -> (w166:T4)
      }
      frame "ConfigureLoadToSinglepoint" {
        w203 = 1027 items=["Automatically after Source Complete"=1025, "On Demand"=1026, "On Measure Trigger"=1027] ("Measurement:Advanced:Measure When")
        w223 = T14 1007 items=["DC Voltage"=1006, "DC Current"=1007, "Pulse Voltage"=1049, "Pulse Current"=1050] ("output function")
        w222 = T9 1020 items=["Single Point"=1020, "Sequence"=1021] ("source mode")
        n68 = Unbundle By Name(w207) -> ("Measure record length smu"=w210:i32, "Aperture time"=w209:dbl)
        n69 = Unbundle By Name(w207) -> ("Load channel name"=w198:string, "Load out"=w229:refnum<k15>)
        n70 = Unbundle By Name(w211) -> ("Load transient response"=w216:i32, "Load current gain bandwidth"=w215:dbl, "Load current compensation frequency"=w214:dbl, "Load current pole-zero ratio"=w212:dbl)
        n71 = Unbundle By Name(w207) -> ("Source terminal name"=w228:string, "Measure load terminal name"=w227:string)
        n72 = call <instrlib>:"niDCPower Configure Source Mode With Channels.vi"("error in (no error)"=w213, "source mode"=w222, "channel name"=w198, "instrument handle"=w229) -> ("error out"=w220:errorcluster, "instrument handle out"=w221:refnum<k15>)  [unwired: 6 in]
        n73 = call <instrlib>:"niDCPower Configure Output Function.vi"("error in (no error)"=w220, "output function"=w223, "channel name"=w198, "instrument handle"=w221) -> ("error out"=w225:errorcluster, "instrument handle out"=w224:refnum<k15>)  [unwired: 6 out]
        n74 = call-poly <instrlib>:"niDCPower Configure Trigger With Channels (Poly).vi"("error in (no error)"=w225, "input terminal"=w228, "channel name"=w198, "instrument handle"=w224) -> ("error out"=w217:errorcluster, "instrument handle out"=w226:refnum<k15>)  [unwired: 6 in]
        n75 = property class="niDCPower"(reference=w226, error in=w217, "Transient Response"=w216, "Current GBW"=w215, "Current Compensation Freq"=w214, "Current Pole-Zero Ratio"=w212, "Measure Record Length"=w210, "Aperture Time"=w209) -> (reference out=w219:refnum<k15>, error out=w218:errorcluster)
        n76 = call-poly <instrlib>:"niDCPower Configure Trigger With Channels (Poly).vi"("error in (no error)"=w218, "input terminal"=w227, "channel name"=w198, "instrument handle"=w219) -> ("error out"=w202:errorcluster, "instrument handle out"=w200:refnum<k15>)  [unwired: 6 in]
        n77 = property class="niDCPower"(reference=w200, error in=w202, "Measure When"=w203) -> (reference out=w199:refnum<k15>, error out=w201:errorcluster)
        n78 = call <instrlib>:"niDCPower Commit With Channels.vi"("error in (no error)"=w201, "channel name"=w198, "instrument handle"=w199) -> ("error out"=w208:errorcluster, "instrument handle out"=w206:refnum<k15>)  [unwired: 7 in]
        n79 = Bundle By Name(cluster=w207, "Load out"=w206) -> (w205:T4)
      }
      frame "ConfigureAndInitiateScope" {
        w237 = 2  # Number of records
        w255 = TRUE  # Enable TClk
        # "Perform scope measurements twice around the rising and falling edges of the source voltage."
        n80 = Unbundle By Name(w234) -> ("Pin Names for Scope"=w238:string[], "vertical range"=w254:dbl[], "vertical offset"=w253:dbl[], "probe attenuation"=w252:dbl[], "vertical coupling"=w251:T2[], "channel enabled"=w250:bool[], "input impedance"=w249:u32[], "max input frequency"=w248:dbl[], "min sample rate"=w247:dbl[], "reference position"=w246:dbl[], "min record length"=w245:i32[], "enforce realtime"=w244:bool[])
        n81 = Unbundle By Name(w231) -> ("Scope ref trigger source"=w239:string)
        n82 = Bundle By Name(cluster=w231, "Number of records"=w237, "Enable TClk"=w255) -> (w241:T4)
        n83 = Array Size(array=w244) -> (size(s)=w243:i32)
        n84 = Initialize Array(w237, w243) -> (w242:i32[])
        n85 = Build Cluster Array(w254, w253, w252, w251, w250, w249, w248, w247, w246, w245, w242, w244) -> (w240:T15)
        n86 = case shown="True" w255 {
          tunnel: w236 -> [w260 w299]
          tunnel: w241 -> [w269 w306]
          tunnel: [w268 w300] -> w230
          tunnel: [w267 w307] -> w235
          tunnel: w233 -> [w261 w298]
          tunnel: [w261 w298] -> w232
          tunnel: w240 -> [w257 w296]
          tunnel: w239 -> [w259 w295]
          tunnel: w238 -> [w258 w297]
          frame False {
            # "TClk has not been supported by grpc-device and cannot be used with the Measurement Plug-In APIs as of 2024 Q4.\nFor strict synchronization with TClk, you need to use the niScope Initialize with Options VI to initialize sessions."
            n87 = Array Size(array=w258) -> (size(s)=w262:i32)
            n88 = case shown="1.." w262 {
              tunnel: w261 -> [_ w282]
              tunnel: w260 -> [w270 w281]
              tunnel: w258 -> [_ w275]
              tunnel: [_ w274] -> w256
              tunnel: [_ w273] -> w265
              tunnel: [w270 w272] -> w264
              tunnel: [_ w271] -> w263
              frame 0, Default {
              }
              frame 1.. {
                n89 = call-poly <vilib>:"Reserve Sessions.vi"("error in"=w281, "pin or relay names"=w275, "measurement context in"=w282) -> ("error out"=w280:errorcluster, "session reservation out"=w279:refnum<class "Session Reservation.lvclass">)  [unwired: 6 in, 1 out]
                n90 = call-poly <vilib>:"Initialize Sessions.vi"("error in"=w280, "reset"=FALSE, "session reservation in"=w279) -> ("error out"=w278:errorcluster, "sessions"=w273:refnum<k15>[], "session reservation out"=w277:refnum<class "Session Reservation.lvclass">)  [unwired: 5 in, 1 out]
                n91 = call-poly <vilib>:"Get Connections.vi"("error in"=w278, "pin or relay names"=w275, "session reservation in"=w277) -> ("error out"=w272:errorcluster, "connections"=w271:T16[], "session reservation out"=w274:refnum<class "Session Reservation.lvclass">)  [unwired: 6 in]
              }
            }
            n92 = Bundle By Name(cluster=w269, "scope session reservation"=w256) -> (w268:T4)
            n93 = for {
              tunnel: w263 -> [w294] mode=indexing
              shift-right: [w287] -> w266
              shift-left: w264 -> [w291]
              tunnel: w259 -> [w288]
              tunnel: w257 -> [w286] mode=indexing
              n94 = Unbundle By Name(w294) -> ("session"=w293:refnum<k15>, "connection.channel"=w292:string)
              n95 = call "Setup Scope.vi"("instrument handle"=w293, "channels"=w292, "Scope Parameters"=w286, "error in"=w291) -> ("instrument handle out"=w289:refnum<k15>, "error out"=w290:errorcluster)  [unwired: 10 in]
              n96 = call-poly <instrlib>:"niScope Configure Trigger (poly).vi"("instrument handle"=w289, "trigger source"=w288, "error in"=w290) -> ("error out"=w287:errorcluster)  [unwired: 11 in, 1 out]
            }
            n97 = for {
              tunnel: w265 -> [w283] mode=indexing
              shift-right: [w284] -> w267
              shift-left: w266 -> [w285]
              n98 = call <instrlib>:"niScope Initiate Acquisition.vi"("instrument handle"=w283, "error in"=w285) -> ("error out"=w284:errorcluster)  [unwired: 12 in, 1 out]
            }
          }
          frame True {
            n99 = call-dynamic "Get Pin Map Context.vi"("error in"=w299, "measure call context in"=w298) -> ("error out"=w310:errorcluster, "pin map context"=w311:T17)  [unwired: 7 in, 1 out]
            n100 = Unbundle By Name(w311) -> ("pin map id"=w309:string)
            n101 = Build Path(name or relative path=w309) -> (appended path=w308:path)  [unwired: 1 in]
            n102 = call "Create Connection Map From Pin Map File.vi"("error in (no error)"=w310, "pin map file path"=w308) -> ("error out"=w303:errorcluster, "connection map"=w305:map{string, T5[]})  [unwired: 8 in]
            n103 = call "Create Scope Info Map for Each Site.vi"("error in (no error)"=w303, "parameters array"=w296, "Pin Names for Scope"=w297, "connection map"=w305) -> ("error out"=w302:errorcluster, "scope info map for each site"=w304:T18)  [unwired: 6 in]
            n104 = for {
              tunnel: w295 -> [w315]
              shift-right: [w314] -> w307
              shift-left: w302 -> [w316]
              tunnel: [w313] -> w301 mode=indexing
              tunnel: w304 -> [w312] mode=indexing
              # "Loop for multiple sites"
              n105 = call "Initialize Configure Initiate Scope with TClk.vi"("error in (no error)"=w316, "ref trigger source"=w315, "scope info map"=w312) -> ("error out"=w314:errorcluster, "scope handles"=w313:refnum<k15>[])  [unwired: 7 in]
            }
            n106 = Bundle By Name(cluster=w306, "connection map"=w305, "instrument info map array"=w304, "Scope handles"=w301) -> (w300:T4)
          }
        }
      }
      frame "StartSourceLoad" {
        n107 = Unbundle By Name(w320) -> ("Source out"=w322:refnum<k15>, "Source channel name"=w323:string, "Load out"=w326:refnum<k15>, "Load channel name"=w327:string)
        n108 = flat-sequence {
          tunnel: [w339] -> w331
          tunnel: [w338] -> w330
          tunnel: [w337] -> w329
          tunnel: w326 -> [w336]
          tunnel: w322 -> [w335]
          tunnel: w323 -> [w332]
          tunnel: w327 -> [w333]
          tunnel: [w332] -> w328
          tunnel: w321 -> [w334]
          tunnel: w331 -> [w346]
          tunnel: w330 -> [w345]
          tunnel: w329 -> [w342]
          tunnel: [w343] -> w324
          tunnel: [w344] -> w318
          tunnel: [w342] -> w325
          tunnel: w328 -> [w341]
          frame #0 {
            n109 = call <instrlib>:"niDCPower Initiate With Channels.vi"("error in (no error)"=w334, "channel name"=w333, "instrument handle"=w336) -> ("error out"=w340:errorcluster, "instrument handle out"=w337:refnum<k15>)  [unwired: 7 in]
            n110 = call <instrlib>:"niDCPower Initiate With Channels.vi"("error in (no error)"=w340, "channel name"=w332, "instrument handle"=w335) -> ("error out"=w338:errorcluster, "instrument handle out"=w339:refnum<k15>)  [unwired: 7 in]
          }
          frame #1 {
            w347 = T8 1033 items=["Source Complete Event"=1030, "Measure Complete Event"=1031, "Sequence Iteration Complete Event"=1032, "Sequence Engine Done Event"=1033] ("event")
            n111 = call <instrlib>:"niDCPower Wait For Event With Channels.vi"("error in (no error)"=w345, "event"=w347, "channel name"=w341, "instrument handle"=w346) -> ("error out"=w344:errorcluster, "instrument handle out"=w343:refnum<k15>)  [unwired: 6 in]
          }
        }
        n112 = Bundle By Name(cluster=w320, "Source out"=w324, "Load out"=w325) -> (w319:T4)
      }
      frame "PerformMeasurement" {
        n113 = Unbundle By Name(w362) -> ("Source out"=w380:refnum<k15>, "Source channel name"=w379:string, "Load out"=w382:refnum<k15>, "Load channel name"=w381:string, "Measure record length smu"=w378:i32)
        n114 = Unbundle By Name(w362) -> ("Number of records"=w363:i32, "Enable TClk"=w370:bool, "scope session reservation"=w369:refnum<class "Session Reservation.lvclass">, "Scope handles"=w366:refnum<k15>[][], "instrument info map array"=w365:T18)
        n115 = Unbundle By Name(w348) -> ("Pin Names for Scope"=w368:string[], "channel enabled"=w367:bool[], "min record length"=w364:i32[])
        n116 = for {
          N: w363 -> [_]
          tunnel: w370 -> [w403]
          tunnel: w369 -> [w402]
          tunnel: w368 -> [w401]
          tunnel: w367 -> [w400]
          tunnel: w364 -> [w399]
          tunnel: w366 -> [w397]
          tunnel: w365 -> [w396]
          tunnel: [w395] -> w360 mode=concatenating
          tunnel: [w394] -> w359 mode=concatenating
          tunnel: [w392] -> w351 mode=concatenating
          shift-right: [w393] -> w354
          shift-left: w361 -> [w398]
          i -> [w391]
          n117 = case shown="True" w403 {
            tunnel: w398 -> [w407 w432]
            tunnel: w399 -> [w404 _]
            tunnel: w391 -> [w405 w429]
            tunnel: [w417 w431] -> w393
            tunnel: [w416 w430] -> w392
            tunnel: w397 -> [_ w433]
            tunnel: w396 -> [_ w428]
            tunnel: [w414 w427] -> w394
            tunnel: [w415 w426] -> w395
            tunnel: w402 -> [w411 _]
            tunnel: w401 -> [w410 _]
            tunnel: w400 -> [w409 _]
            frame False {
              n118 = for {
                tunnel: w410 -> [w425] mode=indexing
                tunnel: w409 -> [w424] mode=indexing
                tunnel: [w425] -> w413 mode=indexing if=w424
              }
              n119 = Array Size(array=w413) -> (size(s)=w412:i32)
              n120 = case shown="1.." w412 {
                tunnel: w407 -> [w418 w423]
                tunnel: [_ w422] -> w406
                tunnel: w411 -> [_ w421]
                tunnel: w413 -> [_ w420]
                tunnel: [w418 w419] -> w408
                frame 0, Default {
                  # "Do nothing if Pin Names are empty."
                }
                frame 1.. {
                  n121 = call-poly <vilib>:"Get Connections.vi"("error in"=w423, "pin or relay names"=w420, "session reservation in"=w421) -> ("error out"=w419:errorcluster, "connections"=w422:T16[])  [unwired: 6 in, 1 out]
                }
              }
              n122 = call "Fetch Waveforms for One Record.vi"("error in (no error)"=w408, "min record length"=w404, "fetch record number"=w405, "connections"=w406) -> ("error out"=w417:errorcluster, "waveforms"=w416:waveform(dbl)[], "sites"=w414:i32[], "pins or relay names"=w415:string[])  [unwired: 4 in]
            }
            frame True {
              n123 = for {
                tunnel: w433 -> [w441] mode=indexing
                shift-right: [w438] -> w431
                shift-left: w432 -> [w440]
                tunnel: [w439] -> w430 mode=concatenating
                tunnel: w429 -> [w437]
                tunnel: w428 -> [w436] mode=indexing
                tunnel: [w435] -> w426 mode=concatenating
                tunnel: [w434] -> w427 mode=concatenating
                # "Loop for multiple sites"
                n124 = call "Fetch Waveforms for One Record with Scope Info Map.vi"("error in (no error)"=w440, "fetch record number"=w437, "scope info map"=w436, "Scope handles"=w441) -> ("error out"=w438:errorcluster, "waverforms"=w439:waveform(dbl)[], "sites"=w434:i32[], "pins"=w435:string[])  [unwired: 4 in]
              }
            }
          }
        }
        n125 = call <instrlib>:"niDCPower Fetch Multiple.vi"("instrument handle"=w380, "channel name"=w379, "count (1)"=w378, "error in (no error)"=w361) -> ("instrument handle out"=w377:refnum<k15>, "voltage measurements"=w375:dbl[], "error out"=w383:errorcluster)  [unwired: 1 in, 8 out]
        n126 = call <instrlib>:"niDCPower Fetch Multiple.vi"("instrument handle"=w382, "channel name"=w381, "count (1)"=w378, "error in (no error)"=w383) -> ("instrument handle out"=w376:refnum<k15>, "voltage measurements"=w374:dbl[], "error out"=w371:errorcluster)  [unwired: 1 in, 8 out]
        n127 = Array Max & Min(array=w374) -> (max value=w373:dbl, min value=w372:dbl)  [unwired: 2 out]
        n128 = call "Concatenate Waveform Array.vi"("waveform array"=w351) -> ("waveform t0 array"=w358:dbl[], "waveform dt array"=w357:dbl[], "waveform length array"=w356:i32[], "concatenated waveform Y"=w355:dbl[])  [unwired: 11 in]
        n129 = Bundle By Name(cluster=w362, "Source out"=w377, "measurement results.Source voltages"=w375, "Load out"=w376, "measurement results.Load voltages"=w374, "measurement results.Overshoot load voltage"=w373, "measurement results.Undershoot load voltage"=w372, "measurement results.waveform pins"=w360, "measurement results.waveform sites"=w359, "measurement results.waveform t0 array"=w358, "measurement results.waveform dt array"=w357, "measurement results.waveform length array"=w356, "measurement results.concatenated waveform Y"=w355) -> (w350:T4)
        n130 = Merge Errors(w371, w354) -> (w353:errorcluster)
        n131 = Unbundle By Name(w350) -> ("measurement results"=w349:T3)
        n132 = disable-structure shown="Disabled" {
          disable-tunnel: w353 -> [w389 w390]
          disable-tunnel: [w388 w390] -> w352
          disable-tunnel: w351 -> [w387 _]
          disable-tunnel: w349 -> [w386 _]
          disable-tunnel: w348 -> [w385 _]
          frame Disabled {
            n133 = call "Save Results to TDMS.vi"("measurement configuration"=w385, "measurement results"=w386, "Scope waveforms"=w387, "error in (no error)"=w389) -> ("error out"=w388:errorcluster)  [unwired: 15 in]
          }
          frame Enabled {
          }
        }
      }
      frame "Exit", Default {
        n134 = Release Queue(queue=w442, error in (no error)=w446) -> (error out=w447:errorcluster)  [unwired: 1 in, 2 out]
        n135 = case shown="Error .." w447 {
          selector: w447 -> [w461 w504]
          tunnel: w444 -> [w460 w505]
          tunnel: [w454 w503] -> w443
          tunnel: w445 -> [w450 w488]
          frame No Error {
            # "Abort, close sessions and updates the status indicator on the operation performed"
            n136 = Unbundle By Name(w460) -> ("Enable TClk"=w453:bool, "Scope handles"=w451:refnum<k15>[][], "scope session reservation"=w452:refnum<class "Session Reservation.lvclass">, "dcpower session reservation"=w456:refnum<class "Session Reservation.lvclass">, "Source out"=w463:refnum<k15>, "Source channel name"=w465:string, "Load out"=w462:refnum<k15>, "Load channel name"=w464:string)
            n137 = call <instrlib>:"niDCPower Abort With Channels.vi"("error in (no error)"=w461, "channel name"=w464, "instrument handle"=w462) -> ("error out"=w466:errorcluster)  [unwired: 7 in, 1 out]
            n138 = call <instrlib>:"niDCPower Abort With Channels.vi"("error in (no error)"=w466, "channel name"=w465, "instrument handle"=w463) -> ("error out"=w458:errorcluster)  [unwired: 7 in, 1 out]
            n139 = call <vilib>:"Close Sessions.vi"("error in"=w458, "session reservation in"=w456) -> ("error out"=w457:errorcluster, "session reservation out"=w459:refnum<class "Session Reservation.lvclass">)  [unwired: 8 in]
            n140 = call <vilib>:"Unreserve Sessions.vi"("error in"=w457, "session reservation in"=w459) -> ("error out"=w455:errorcluster)  [unwired: 9 in]
            n141 = case shown="False" w453 {
              tunnel: w455 -> [w472 w480]
              tunnel: [w471 w479] -> w454
              tunnel: w452 -> [w470 _]
              tunnel: w450 -> [w469 _]
              tunnel: w451 -> [_ w481]
              frame False {
                n142 = Unbundle By Name(w469) -> ("Pin Names for Scope"=w468:string[])
                n143 = Array Size(array=w468) -> (size(s)=w467:i32)
                n144 = case shown="1.." w467 {
                  tunnel: w472 -> [w473 w477]
                  tunnel: [w473 w475] -> w471
                  tunnel: w470 -> [_ w474]
                  frame 0, Default {
                  }
                  frame 1.. {
                    n145 = call <vilib>:"Close Sessions.vi"("error in"=w477, "session reservation in"=w474) -> ("error out"=w476:errorcluster, "session reservation out"=w478:refnum<class "Session Reservation.lvclass">)  [unwired: 8 in]
                    n146 = call <vilib>:"Unreserve Sessions.vi"("error in"=w476, "session reservation in"=w478) -> ("error out"=w475:errorcluster)  [unwired: 9 in]
                  }
                }
              }
              frame True {
                n147 = for {
                  tunnel: w481 -> [w484] mode=indexing
                  shift-right: [w482] -> w479
                  shift-left: w480 -> [w483]
                  n148 = for {
                    tunnel: w484 -> [w485] mode=indexing
                    shift-right: [w486] -> w482
                    shift-left: w483 -> [w487]
                    n149 = call <instrlib>:"niScope Close.vi"("instrument handle"=w485, "error in"=w487) -> ("error out"=w486:errorcluster)  [unwired: 13 in]
                  }
                }
              }
            }
          }
          frame Error {
            # "Resets the device with default values whenever there is an error"
            n150 = Unbundle By Name(w505) -> ("Enable TClk"=w489:bool, "Scope handles"=w490:refnum<k15>[][], "scope session reservation"=w491:refnum<class "Session Reservation.lvclass">, "dcpower session reservation"=w494:refnum<class "Session Reservation.lvclass">, "Source out"=w500:refnum<k15>, "Source channel name"=w499:string, "Load out"=w502:refnum<k15>, "Load channel name"=w501:string)
            n151 = call <instrlib>:"niDCPower Abort With Channels.vi"("channel name"=w501, "instrument handle"=w502) -> ("error out"=w506:errorcluster, "instrument handle out"=w509:refnum<k15>)  [unwired: 8 in]
            n152 = call <instrlib>:"niDCPower Reset With Channels.vi"("error in (no error)"=w506, "channel name"=w501, "instrument handle"=w509) -> ("error out"=w498:errorcluster)  [unwired: 7 in, 1 out]
            n153 = call <instrlib>:"niDCPower Abort With Channels.vi"("error in (no error)"=w498, "channel name"=w499, "instrument handle"=w500) -> ("error out"=w508:errorcluster, "instrument handle out"=w507:refnum<k15>)  [unwired: 7 in]
            n154 = call <instrlib>:"niDCPower Reset With Channels.vi"("error in (no error)"=w508, "channel name"=w499, "instrument handle"=w507) -> ("error out"=w496:errorcluster)  [unwired: 7 in, 1 out]
            n155 = call <vilib>:"Close Sessions.vi"("error in"=w496, "session reservation in"=w494) -> ("error out"=w495:errorcluster, "session reservation out"=w497:refnum<class "Session Reservation.lvclass">)  [unwired: 8 in]
            n156 = call <vilib>:"Unreserve Sessions.vi"("error in"=w495, "session reservation in"=w497) -> ("error out"=w493:errorcluster)  [unwired: 9 in]
            n157 = case shown="False" w489 {
              tunnel: w493 -> [w515 w523]
              tunnel: [w514 w522] -> w492
              tunnel: w491 -> [w513 _]
              tunnel: w488 -> [w512 _]
              tunnel: w490 -> [_ w524]
              frame False {
                n158 = Unbundle By Name(w512) -> ("Pin Names for Scope"=w511:string[])
                n159 = Array Size(array=w511) -> (size(s)=w510:i32)
                n160 = case shown="1.." w510 {
                  tunnel: w515 -> [w516 w520]
                  tunnel: [w516 w518] -> w514
                  tunnel: w513 -> [_ w517]
                  frame 0, Default {
                  }
                  frame 1.. {
                    n161 = call <vilib>:"Close Sessions.vi"("error in"=w520, "session reservation in"=w517) -> ("error out"=w519:errorcluster, "session reservation out"=w521:refnum<class "Session Reservation.lvclass">)  [unwired: 8 in]
                    n162 = call <vilib>:"Unreserve Sessions.vi"("error in"=w519, "session reservation in"=w521) -> ("error out"=w518:errorcluster)  [unwired: 9 in]
                  }
                }
              }
              frame True {
                n163 = for {
                  tunnel: w524 -> [w527] mode=indexing
                  shift-right: [w525] -> w522
                  shift-left: w523 -> [w526]
                  n164 = for {
                    tunnel: w527 -> [w528] mode=indexing
                    shift-right: [w529] -> w525
                    shift-left: w526 -> [w530]
                    n165 = call <instrlib>:"niScope Close.vi"("instrument handle"=w528, "error in"=w530) -> ("error out"=w529:errorcluster)  [unwired: 13 in]
                  }
                }
              }
            }
            n166 = Merge Errors(w504, w492) -> (w503:errorcluster)
          }
        }
      }
    }
  }
  "error out" <- w7
  "measure call context out" <- w4
  n167 = Unbundle By Name(w6) -> ("measurement results"=→"measurement results":T3)
